vi "Stop.vi"() -> ()   [LabVIEW 2012]
panel:
  in  "ֹͣ":bool
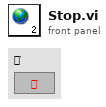
[diagram p1: front panel]
diagram:
